vi "Find val prox.vi"(10 "X":dbl, 11 "Array":dbl[](array[numeric])) -> (3 "Index":i32)   [LabVIEW 2012]
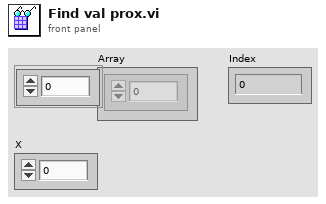
[diagram p1: front panel]
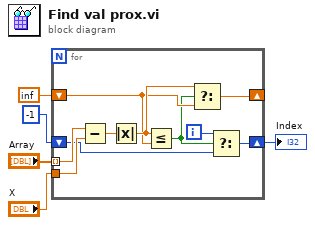
[diagram p0: block diagram]
diagram:
  n1 = for {
    tunnel: "Array" -> [w15] mode=indexing
    tunnel: "X" -> [w14]
    shift-right: [w10] -> _
    shift-left: inf -> [w11]
    shift-right: [w7] -> w5
    shift-left: -1 -> [w6]
    i -> [w8]
    n2 = Subtract(x=w15, y=w14) -> (x-y=w13:dbl)
    n3 = Absolute Value(x=w13) -> (abs(x)=w12:dbl)
    n4 = Less Or Equal?(x=w12, y=w11) -> (x <= y?=w9:bool)
    n5 = Select(t=w12, s=w9, f=w11) -> (s? t:f=w10:dbl)
    n6 = Select(t=w8, s=w9, f=w6) -> (s? t:f=w7:i32)
  }
  "Index" <- w5
